vi "Get newest file in folder.vi"(8 "error in (no error)":errorcluster, 11 "Target folder":path=path "L:/junk") -> (0 "error out":errorcluster, 2 "filenames":string[](array[string]), 3 "Newest file pathname":path)   [LabVIEW 2013]
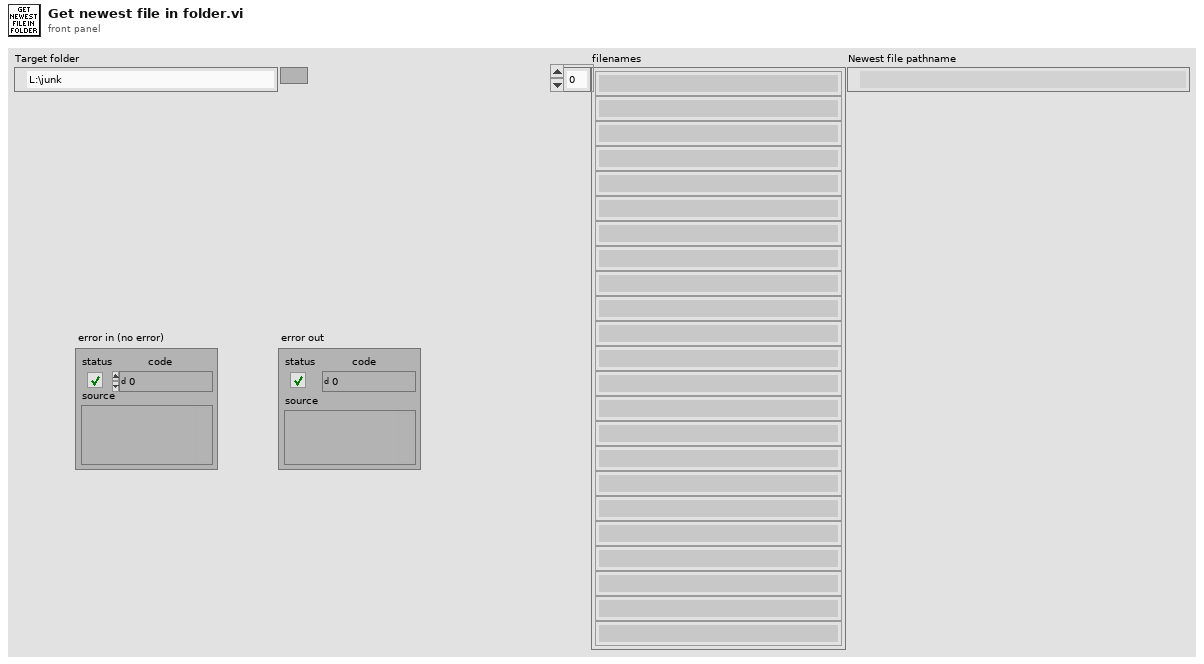
[diagram p1: front panel]
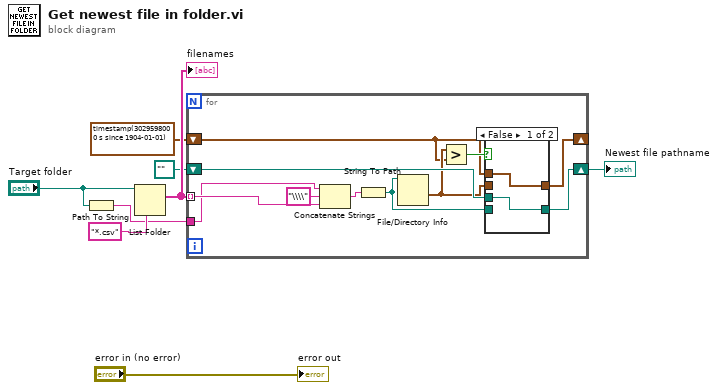
[diagram p0: block diagram]
diagram:
  n1 = Path To String(path="Target folder") -> (string=w2:string)
  n2 = List Folder(path="Target folder", pattern="*.csv") -> (filenames=w7:string[])  [unwired: 2 in, 3 out]
  "filenames" <- w7
  n3 = for {
    tunnel: w7 -> [w19] mode=indexing
    shift-right: [w13] -> _
    shift-left: timestamp(3029598000 s since 1904-01-01) -> [w11]
    shift-right: [w14] -> w4
    shift-left: path "" ("path") -> [w16]
    tunnel: w2 -> [w10]
    n4 = Concatenate Strings(w10, "\\\\" ("string"), w19) -> (w18:string)
    n5 = String To Path(string=w18) -> (path=w15:path)
    n6 = File/Directory Info(path=w15) -> (last mod=w12:timestamp)  [unwired: 1 in, 6 out]
    n7 = Greater?(x=w12, y=w11) -> (0:w17:bool)
    n8 = case shown="False" w17 {
      tunnel: w16 -> [w21 _]
      tunnel: w15 -> [_ w23]
      tunnel: [w21 w23] -> w14
      tunnel: [w20 w22] -> w13
      tunnel: w12 -> [_ w22]
      tunnel: w11 -> [w20 _]
      frame False {
      }
      frame True {
      }
    }
  }
  "Newest file pathname" <- w4
  "error out" <- "error in (no error)"
